vi "Set Value.vi"(8 "error in":errorcluster, 10 "Value":variant, 11 "Image in":refnum<class "Image.lvclass">) -> (0 "error out":errorcluster, 3 "Image out":refnum<class "Image.lvclass">)   [LabVIEW 2024, in "SourceGrid.lvlib" / "Image.lvclass"]
uses:
  Image.lvclass
  System.Drawing
  D:/git/Sourcegrid-LabVIEW/dll/SourceGrid.dll
  dll/SourceGrid.dll
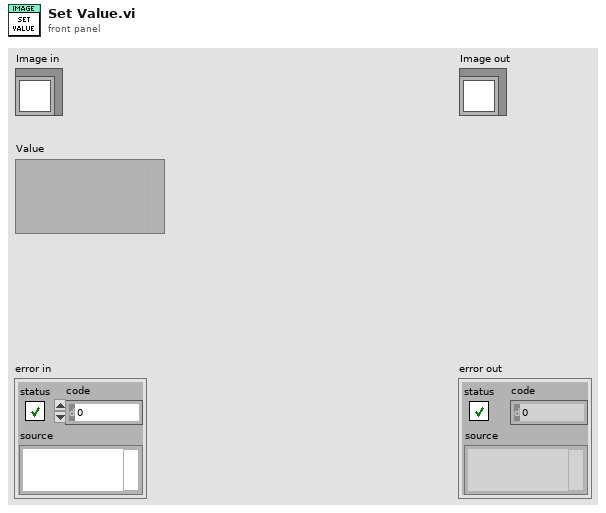
[diagram p1: front panel]
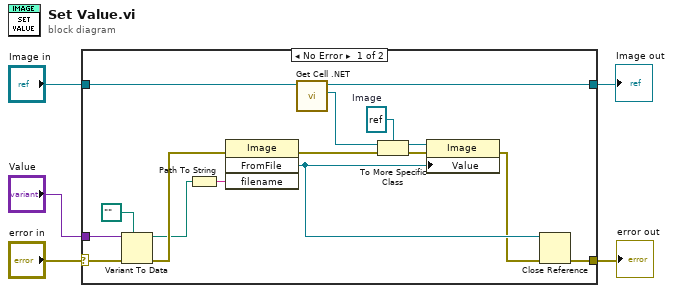
[diagram p0: block diagram]
diagram:
  n1 = case shown="No Error" "error in" {
    selector: "error in" -> [w16 w23]
    tunnel: [w8 w23] -> w4
    tunnel: "Image in" -> [w15 w22]
    tunnel: [w14 w22] -> w2
    tunnel: "Value" -> [w13 _]
    frame No Error {
      w11 = refnum<k24> refnum  # Image
      n2 = Variant To Data(error in=w16, type=path "", Variant=w13) -> (data=w17:path, error out=w19:errorcluster)
      n3 = Path To String(path=w17) -> (string=w20:string)
      n4 = invoke class="Image" method="FromFile"(error in=w19, "filename"=w20) -> (error out=w21:errorcluster, "FromFile"=w10:refnum<k24>)  [unwired: 2 in, 2 out]
      n5 = call-dynamic "Get Cell .NET.vi"("Cell in"=w15) -> ("Cell .NET"=w12:refnum<k24>, "Cell out"=w14:refnum<class "Image.lvclass">)  [unwired: 9 in]
      n6 = To More Specific Class(target class=w11, reference=w12, error in=w21) -> (specific class reference=w7:refnum<k24>, error out=w6:errorcluster)
      n7 = property class="Image"(reference=w7, error in=w6, "Value"=w10) -> (error out=w9:errorcluster)  [unwired: 1 out]
      n8 = Close Reference(reference=w10, error in (no error)=w9) -> (error out=w8:errorcluster)
    }
    frame Error {
    }
  }
  "error out" <- w4
  "Image out" <- w2
